vi "Draw Node Arrow.vi"(7 "Point":cluster{"x":i16, "y":i16}, 10 "Action Diagram In":picture) -> (2 "Action Diagram":picture)   [LabVIEW 2022 SP3, in "FlexBlocks Support.lvlib"]
uses:
  FlexBlocks Support.lvlib
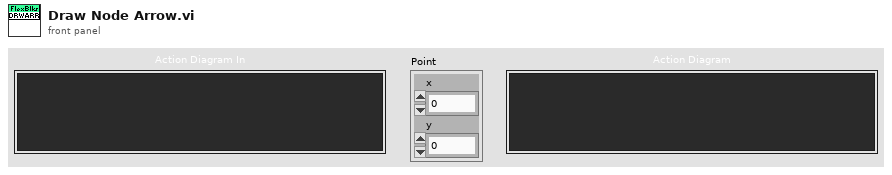
[diagram p1: front panel]
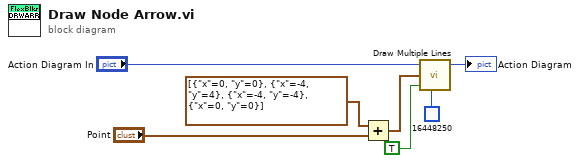
[diagram p0: block diagram]
diagram:
  n1 = Add(x=cluster{"x":i16, "y":i16}[] [{"x"=0, "y"=0}, {"x"=-4, "y"=4}, {"x"=-4, "y"=-4}, {"x"=0, "y"=0}] ("line endpoints"), y="Point") -> (x+y=w5:cluster{"x":i16, "y":i16}[])
  n2 = call <vilib>:"Draw Multiple Lines.vi"("picture"="Action Diagram In", "line endpoints"=w5, "fill?(F)"=TRUE, "color(black)"=u32 16448250) -> ("new picture"=→"Action Diagram":picture)  [unwired: 5 in]
